vi "FG_PowerHandle.vi"(7 "Enum":T1, 8 "error in (no error)":errorcluster, 11 "Handle in":u32) -> (0 "error out":errorcluster, 3 "Handle out":u32)   [LabVIEW 2020]
doc: "Power request handle\n(prevent sytem hybernate FG)"
uses:
  Power Availabilty Requests/Type Defs/Test_PR_typedef.ctl
  Builds/Sgraph_lib_V1.lvlib
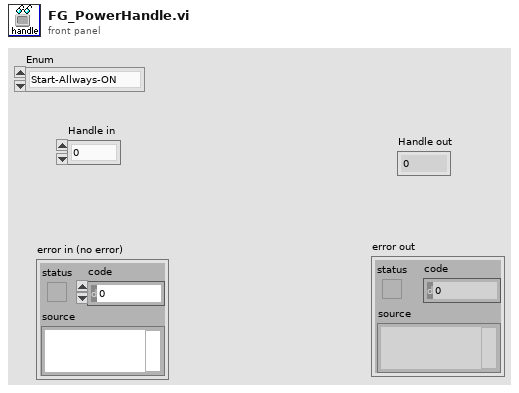
[diagram p1: front panel]
types:
  T1 = typedef "Sgraph_lib_V1.lvlib/Test_PR_typedef.ctl" = enum16{"Start-Allways-ON", "Read-handle"}
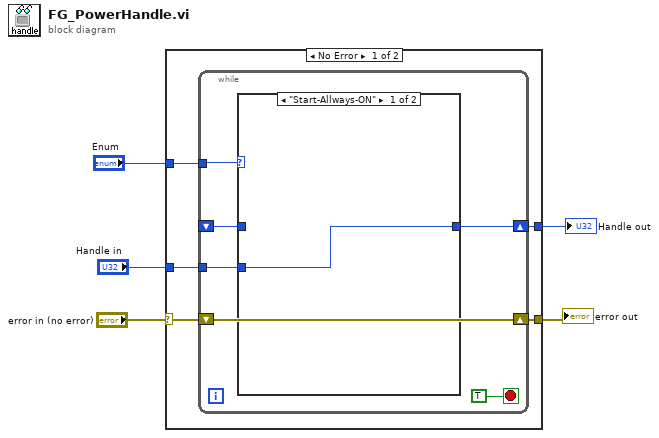
[diagram p0: block diagram]
diagram:
  n1 = case shown="No Error" "error in (no error)" {
    selector: "error in (no error)" -> [w7 w20]
    tunnel: "Handle in" -> [w9 w19]
    tunnel: "Enum" -> [w10 _]
    tunnel: [w8 w19] -> w2
    tunnel: [w6 w20] -> w1
    frame No Error {
      n2 = while {
        tunnel: w10 -> [w15]
        shift-right: [w12] -> w8
        shift-left: _ -> [w14]
        tunnel: w9 -> [w13]
        shift-right: [w11] -> w6
        shift-left: w7 -> [w11]
        stop <- TRUE stop-if-true
        n3 = case shown="\"Start-Allways-ON\"" w15 {
          tunnel: w14 -> [_ w18]
          tunnel: w13 -> [w17 _]
          tunnel: [w17 w18] -> w12
          frame "Start-Allways-ON" {
          }
          frame "Read-handle", Default {
          }
        }
      }
    }
    frame Error {
    }
  }
  "error out" <- w1
  "Handle out" <- w2
